vi "Loop Multiple.vi"(1 "millisecond multiple":u32, 2 "Iteration":i32=1) -> ()   [LabVIEW 2015]
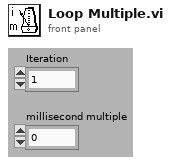
[diagram p1: front panel]
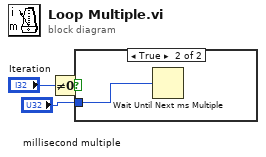
[diagram p0: block diagram]
diagram:
  n1 = Not Equal To 0?(x="Iteration") -> (x != 0?=w1:bool)
  n2 = case shown="True" w1 {
    tunnel: "millisecond multiple" -> [_ w4]
    frame False {
    }
    frame True {
      n3 = Wait Until Next ms Multiple(millisecond multiple=w4) -> ()  [unwired: 1 out]
    }
  }
